vi "CRYDIN data.vi"() -> (3 "Upper Slopes1":dbl[][](array[numeric]), 4 "lowFrequeccy Threshold":dbl[](array[numeric]), 6 "thresholdin quiet1":dbl[](array[numeric]), 8 "OutEar Transmission1":dbl[](array[numeric]), 10 "Slope Threshold1":dbl[](array[numeric]), 13 "UpperLimit of CriticalBands1":dbl[](array[numeric]), 14 "CriticalBandCorrection1":dbl[](array[numeric]), 15 "diffuseFieldCorrection1":dbl[](array[numeric]))   [LabVIEW 2013]
panel:
  out "LowFrequencyCorrection":dbl[][](array[numeric])
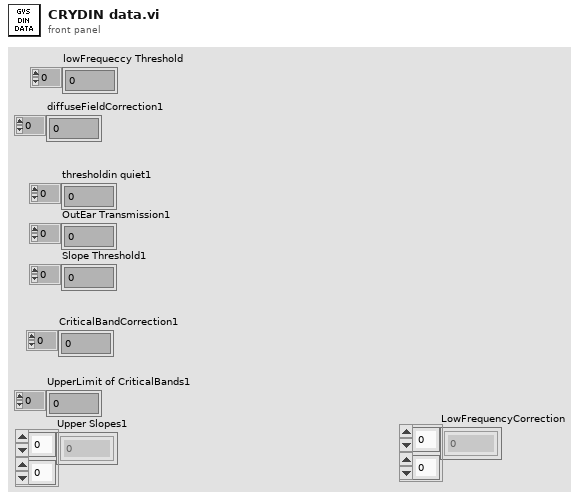
[diagram p1: front panel]
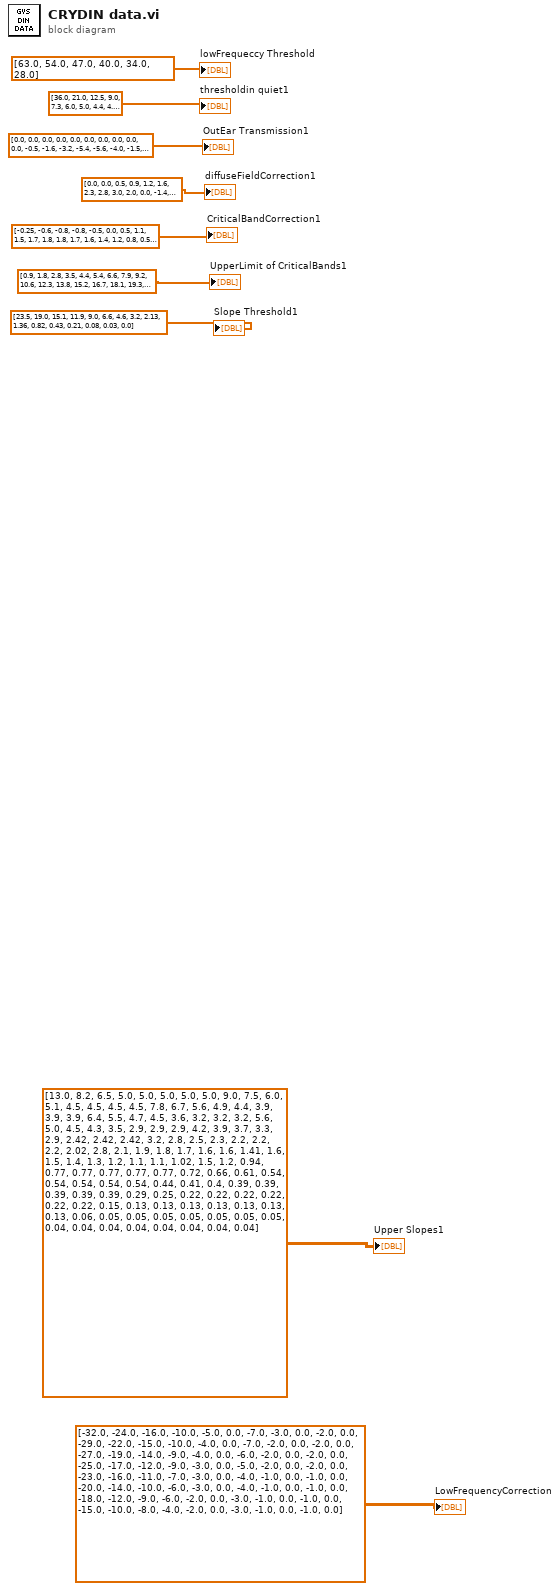
[diagram p0: block diagram]
diagram:
  "lowFrequeccy Threshold" <- dbl[] [63.0, 54.0, 47.0, 40.0, 34.0, 28.0]
  "thresholdin quiet1" <- dbl[] [36.0, 21.0, 12.5, 9.0, 7.3, 6.0, 5.0, 4.4, 4.0, 4.0, 4.0, 4.0, 4.0, 4.0, 4.0, 4.0, 4.0, 4.0, 4.0, 4.0, 0.0]
  "OutEar Transmission1" <- dbl[] [0.0, 0.0, 0.0, 0.0, 0.0, 0.0, 0.0, 0.0, 0.0, 0.0, -0.5, -1.6, -3.2, -5.4, -5.6, -4.0, -1.5, 2.0, 5.0, 12.0]
  "diffuseFieldCorrection1" <- dbl[] [0.0, 0.0, 0.5, 0.9, 1.2, 1.6, 2.3, 2.8, 3.0, 2.0, 0.0, -1.4, -2.0, -1.9, -1.0, 0.5, 3.0, 4.0, 4.3, 4.0]
  "CriticalBandCorrection1" <- dbl[] [-0.25, -0.6, -0.8, -0.8, -0.5, 0.0, 0.5, 1.1, 1.5, 1.7, 1.8, 1.8, 1.7, 1.6, 1.4, 1.2, 0.8, 0.5, 0.0, -0.5]
  "UpperLimit of CriticalBands1" <- dbl[] [0.9, 1.8, 2.8, 3.5, 4.4, 5.4, 6.6, 7.9, 9.2, 10.6, 12.3, 13.8, 15.2, 16.7, 18.1, 19.3, 20.6, 21.8, 22.7, 23.6, 24.0]
  "Slope Threshold1" <- dbl[] [23.5, 19.0, 15.1, 11.9, 9.0, 6.6, 4.6, 3.2, 2.13, 1.36, 0.82, 0.43, 0.21, 0.08, 0.03, 0.0]
  "Upper Slopes1" <- dbl[][] [[13.0, 8.2, 6.5, 5.0, 5.0, 5.0, 5.0, 5.0], [9.0, 7.5, 6.0, 5.1, 4.5, 4.5, 4.5, 4.5], [7.8, 6.7, 5.6, 4.9, 4.4, 3.9, 3.9, 3.9], [6.4, 5.5, 4.7, 4.5, 3.6, 3.2, 3.2, 3.2], [5.6, 5.0, 4.5, 4.3, 3.5, 2.9, 2.9, 2.9], [4.2, 3.9, 3.7, 3.3, 2.9, 2.42, 2.42, 2.42], [3.2, 2.8, 2.5, 2.3, 2.2, 2.2, 2.2, 2.02], [2.8, 2.1, 1.9, 1.8, 1.7, 1.6, 1.6, 1.41], [1.6, 1.5, 1.4, 1.3, 1.2, 1.1, 1.1, 1.02], [1.5, 1.2, 0.94, 0.77, 0.77, 0.77, 0.77, 0.77], [0.72, 0.66, 0.61, 0.54, 0.54, 0.54, 0.54, 0.54], [0.44, 0.41, 0.4, 0.39, 0.39, 0.39, 0.39, 0.39], [0.29, 0.25, 0.22, 0.22, 0.22, 0.22, 0.22, 0.22], [0.15, 0.13, 0.13, 0.13, 0.13, 0.13, 0.13, 0.13], [0.06, 0.05, 0.05, 0.05, 0.05, 0.05, 0.05, 0.05], [0.04, 0.04, 0.04, 0.04, 0.04, 0.04, 0.04, 0.04]]
  "LowFrequencyCorrection" <- dbl[][] [[-32.0, -24.0, -16.0, -10.0, -5.0, 0.0, -7.0, -3.0, 0.0, -2.0, 0.0], [-29.0, -22.0, -15.0, -10.0, -4.0, 0.0, -7.0, -2.0, 0.0, -2.0, 0.0], [-27.0, -19.0, -14.0, -9.0, -4.0, 0.0, -6.0, -2.0, 0.0, -2.0, 0.0], [-25.0, -17.0, -12.0, -9.0, -3.0, 0.0, -5.0, -2.0, 0.0, -2.0, 0.0], [-23.0, -16.0, -11.0, -7.0, -3.0, 0.0, -4.0, -1.0, 0.0, -1.0, 0.0], [-20.0, -14.0, -10.0, -6.0, -3.0, 0.0, -4.0, -1.0, 0.0, -1.0, 0.0], [-18.0, -12.0, -9.0, -6.0, -2.0, 0.0, -3.0, -1.0, 0.0, -1.0, 0.0], [-15.0, -10.0, -8.0, -4.0, -2.0, 0.0, -3.0, -1.0, 0.0, -1.0, 0.0]]
